vi "simpleInterpreter.vi"() -> ()   [LabVIEW 2011]
uses:
  <vilib>/Utility/inputDevices.llb/keyboardAcquire.vi
panel:
  out "error out":errorcluster
  out "lua_State *L":u64
  out "lua_State *print thread":u64
  in  "status refrash":bool
  in  "command refrash":bool
  out "stack":i32
  out "LoadBufferStatus":i32(ring) items=["LUA_OK", "LUA_YIELD", "LUA_ERRRUN", "LUA_ERRSYNTAX", "LUA_ERRMEM", "LUA_ERRGCMM", "LUA_ERRERR"]
  out "PcallStatus":i32(ring) items=["LUA_OK", "LUA_YIELD", "LUA_ERRRUN", "LUA_ERRSYNTAX", "LUA_ERRMEM", "LUA_ERRGCMM", "LUA_ERRERR"]
  in  "停止":bool
  in  "command(ctrl+enter)":string
  out "status":string
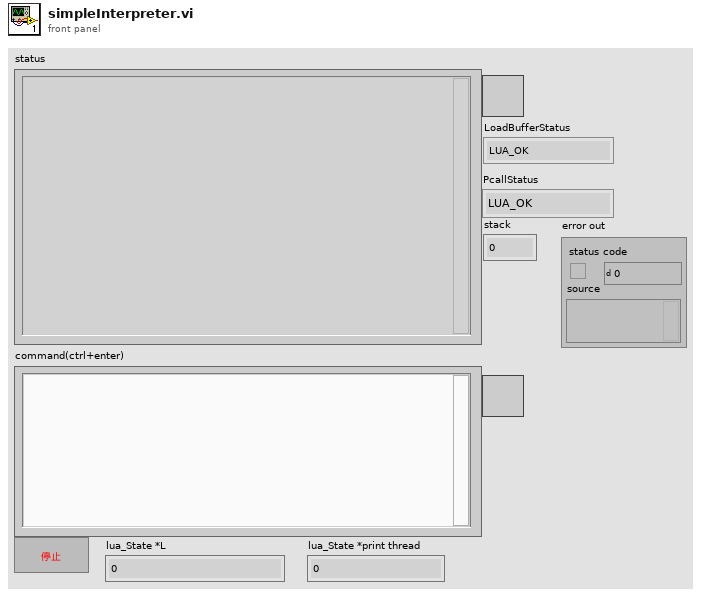
[diagram p1: front panel]
types:
  T1 = enum16{"0", "1", "2", "3", "4", "5", "6", "7", "8", "9", "A", "B", "C", "D", "E", "F", "G", "H", "I", "J", "K", "L", "M", "N", "O", "P", "Q", "R", "S", "T", "U", "V", "W", "X", "Y", "Z", "F1", "F2", "F3", "F4", "F5", "F6", "F7", "F8", "F9", "F10", "F11", "F12", "F13", "F14", "F15", "ADD", "BACK", "BACKSLASH", "CAPITAL", "COMMA", "DECIMAL", "DELETE", "DIVIDE", "DOWN", "END", "EQUALS", "ESCAPE", "GRAVE (`)", "HOME", "INSERT", "LBRACKET", "LCONTROL", "LEFT", "L ALT", "LSHIFT", "LWIN", "MINUS", "MULTIPLY", "NEXT", "NUMLOCK", "NUMPAD_0", "NUMPAD_1", "NUMPAD_2", "NUMPAD_3", "NUMPAD_4", "NUMPAD_5", "NUMPAD_6", "NUMPAD_7", "NUMPAD_8", "NUMPAD_9", "PAUSE", "PERIOD", "PRIOR (PG UP)", "RBRACKET", "RCONTROL", "RETURN", "RIGHT", "R ALT", "RSHIFT", "RWIN", "SCROLL", "SEMICOLON", "SLASH", "SPACE", "SUBTRACT", "TAB", "UP", "ENTER (num pad)", "' (quote)"}[]
  T2 = enum16{"0", "1", "2", "3", "4", "5", "6", "7", "8", "9", "A", "B", "C", "D", "E", "F", "G", "H", "I", "J", "K", "L", "M", "N", "O", "P", "Q", "R", "S", "T", "U", "V", "W", "X", "Y", "Z", "F1", "F2", "F3", "F4", "F5", "F6", "F7", "F8", "F9", "F10", "F11", "F12", "F13", "F14", "F15", "ADD", "BACK", "BACKSLASH", "CAPITAL", "COMMA", "DECIMAL", "DELETE", "DIVIDE", "DOWN", "END", "EQUALS", "ESCAPE", "GRAVE (`)", "HOME", "INSERT", "LBRACKET", "LCONTROL", "LEFT", "L ALT", "LSHIFT", "LWIN", "MINUS", "MULTIPLY", "NEXT", "NUMLOCK", "NUMPAD_0", "NUMPAD_1", "NUMPAD_2", "NUMPAD_3", "NUMPAD_4", "NUMPAD_5", "NUMPAD_6", "NUMPAD_7", "NUMPAD_8", "NUMPAD_9", "PAUSE", "PERIOD", "PRIOR (PG UP)", "RBRACKET", "RCONTROL", "RETURN", "RIGHT", "R ALT", "RSHIFT", "RWIN", "SCROLL", "SEMICOLON", "SLASH", "SPACE", "SUBTRACT", "TAB", "UP", "ENTER (num pad)", "' (quote)"}
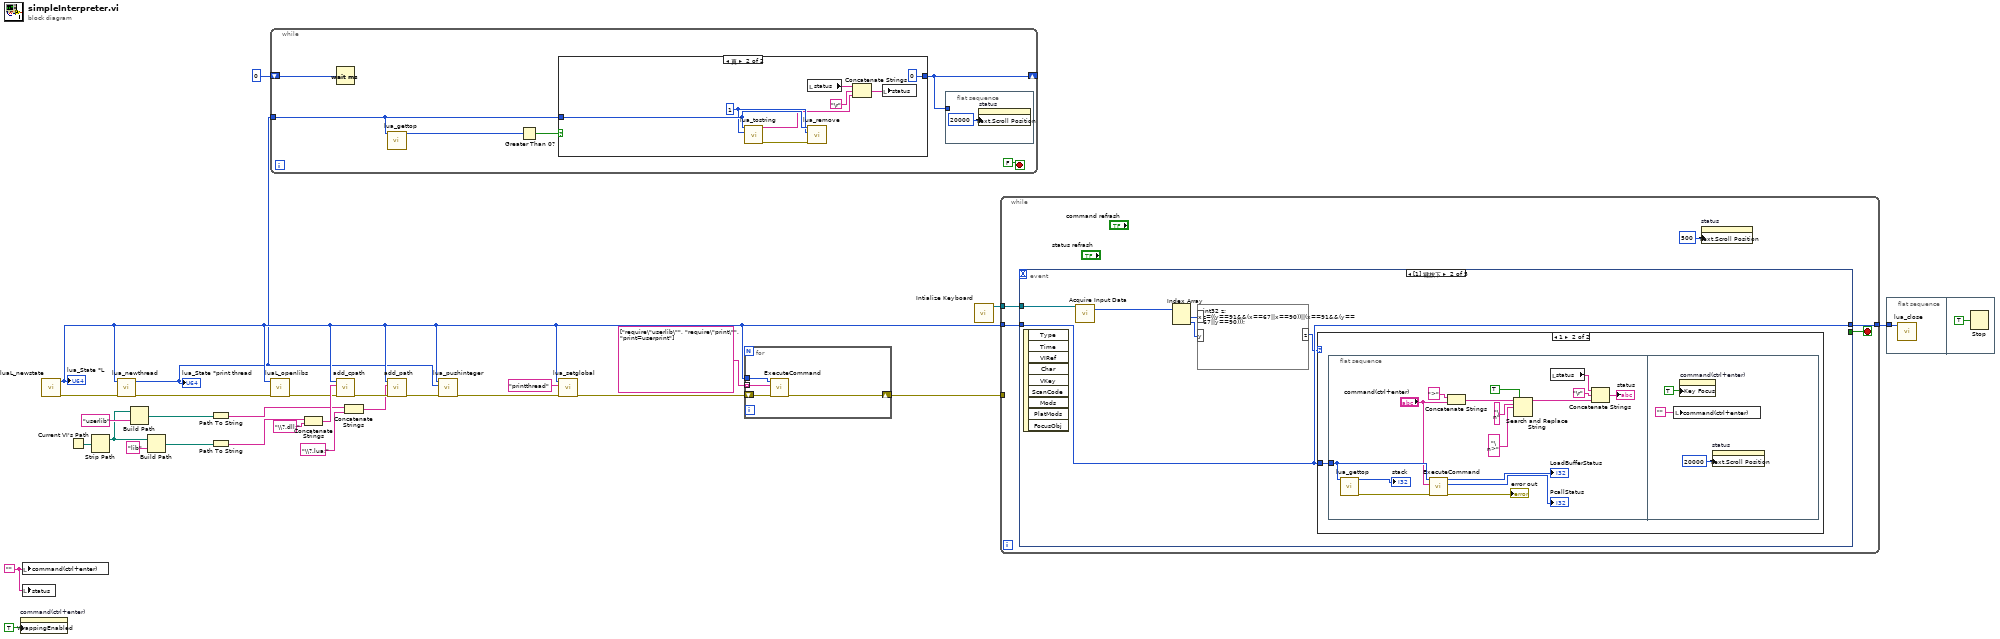
[diagram p0: block diagram]
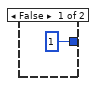
[diagram p2: hidden frame]
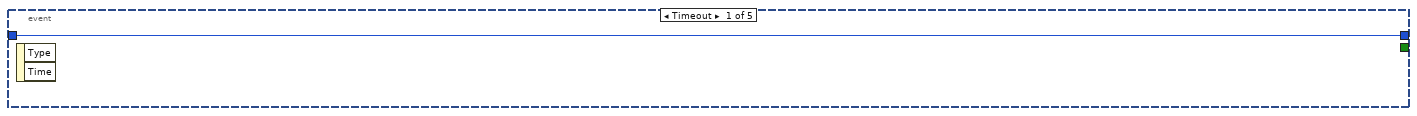
[diagram p3: hidden frame]
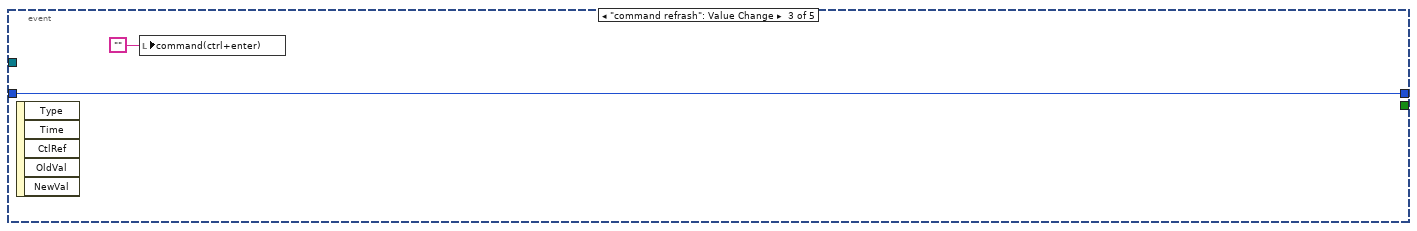
[diagram p5: hidden frame]
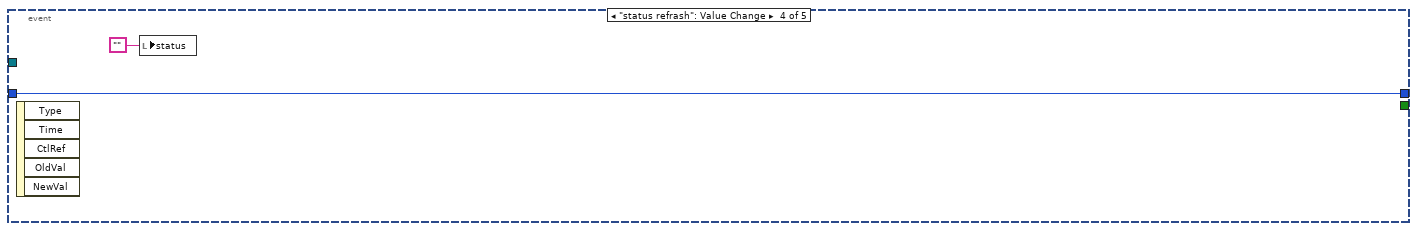
[diagram p6: hidden frame]
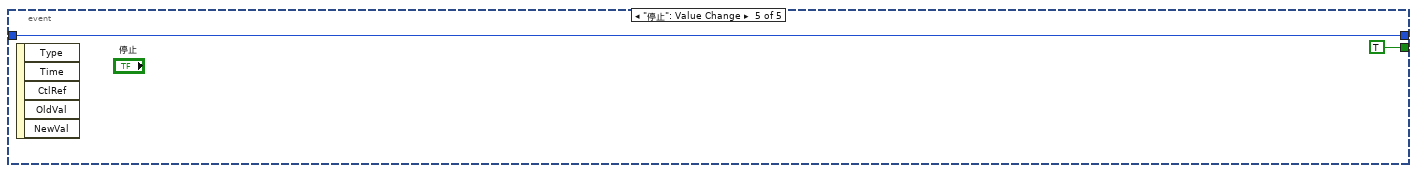
[diagram p7: hidden frame]
diagram:
  w29 = ""
  n1 = property on="command(ctrl+enter)" class="Str"("WrappingEnabled"=TRUE ("启用自动换行")) -> ()  [unwired: 2 in, 2 out]
  n2 = local write "command(ctrl+enter)"(w29) -> ()
  n3 = local write "status"(w29) -> ()
  n4 = call "luaL_newstate.vi"() -> ("error out"=w13:errorcluster, "lua_State *luaL_newstate"=w5:u64)  [unwired: 10 in]
  "lua_State *L" <- w5
  n5 = Current VI's Path() -> (path=w26:path)
  n6 = Strip Path(path=w26) -> (stripped path=w17:path)  [unwired: 1 out]
  n7 = call "lua_newthread.vi"("error in"=w13, "lua_State *L"=w5) -> ("error out"=w12:errorcluster, "lua_State *lua_newthread"=w2:u64)  [unwired: 8 in]
  "lua_State *print thread" <- w2
  n8 = Build Path(base path=w17, name or relative path="userlib" ("名称或相对路径")) -> (appended path=w24:path)
  n9 = Build Path(base path=w17, name or relative path="lib" ("名称或相对路径")) -> (appended path=w15:path)
  n10 = Path To String(path=w24) -> (string=w19:string)
  n11 = Path To String(path=w15) -> (string=w14:string)
  n12 = while {
    tunnel: w2 -> [w33]
    shift-right: [w30] -> _
    shift-left: u32 0 ("等待时间（毫秒）") -> [w31]
    stop <- FALSE stop-if-true
    n13 = Wait (ms)(milliseconds to wait=w31) -> ()  [unwired: 1 out]
    n14 = call "lua_gettop.vi"("lua_State *L"=w33) -> ("lua_gettop"=w34:i32)  [unwired: 9 in, 1 out]
    n15 = Greater Than 0?(x=w34) -> (x > 0?=w32:bool)
    n16 = case shown="真" w32 {
      tunnel: w33 -> [_ w43]
      tunnel: [u32 1 ("等待时间（毫秒）") u32 0 ("等待时间（毫秒）")] -> w30
      frame False {
      }
      frame True {
        w42 = 1 ("index")
        n17 = call "lua_tostring.vi"("index"=w42, "lua_State *L"=w43) -> ("error out"=w44:errorcluster, "constant string"=w38:string)  [unwired: 8 in]
        n18 = local read "status"() -> (w40:string)
        n19 = call "lua_remove.vi"("error in"=w44, "int index"=w42, "lua_State *L"=w43) -> ()  [unwired: 8 in, 1 out]
        n20 = Concatenate Strings(w40, "\r", w38) -> (w41:string)
        n21 = local write "status"(w41) -> ()
      }
    }
    n22 = flat-sequence {
      tunnel: w30 -> [_]
      frame #0 {
        n23 = property on="status" class="Str"("Text.Scroll Position"=u32 20000 ("文本.滚动条位置")) -> ()  [unwired: 2 in, 2 out]
      }
    }
  }
  n24 = call "luaL_openlibs.vi"("error in"=w12, "lua_State *L"=w5) -> ("error out"=w11:errorcluster)  [unwired: 9 in]
  n25 = Concatenate Strings(w14, "\\?.dll;" ("字符串")) -> (w22:string)
  n26 = call "add_cpath.vi"("error in"=w11, "string"=w22, "lua_State *L"=w5) -> ("error out"=w21:errorcluster)  [unwired: 8 in]
  n27 = Concatenate Strings(w19, "\\?.lua;" ("字符串")) -> (w18:string)
  n28 = call "add_path.vi"("error in"=w21, "string"=w18, "lua_State *L"=w5) -> ("error out"=w7:errorcluster)  [unwired: 8 in]
  n29 = call "lua_pushinteger.vi"("error in"=w7, "lua_Integer n"=w2, "lua_State *L"=w5) -> ("error out"=w6:errorcluster)  [unwired: 8 in]
  n30 = call "lua_setglobal.vi"("error in"=w6, "s"="printthread" ("const char *k"), "lua_State *L"=w5) -> ("error out"=w3:errorcluster)  [unwired: 8 in]
  n31 = for {
    shift-right: [w48] -> w9
    shift-left: w3 -> [w49]
    tunnel: w5 -> [w47]
    tunnel: string[] ["require\"userlib\"", "require\"print\"", "print=userprint"] -> [w46] mode=indexing
    n32 = call "ExecuteCommand.vi"("error in"=w49, "command(ctrl+enter)"=w46, "lua_State *luaL_newstate"=w47) -> ("error out"=w48:errorcluster)  [unwired: 6 in, 2 out]
  }
  n33 = call <vilib>:"Intialize Keyboard.vi"() -> ("device ID"=w27:refnum<k1>)  [unwired: 10 in, 1 out]
  n34 = while {
    tunnel: w5 -> [w54]
    tunnel: [w52] -> w1
    tunnel: w27 -> [w51]
    tunnel: w9 -> [_]
    stop <- w53 stop-if-true
    n35 = event shown="[1] 键按下" {
      selector: _ -> [_ _ _ _ _]
      dyn-events: _ -> [_ _ _ _ _]
      timeout: _ -> [_ _ _ _ _]
      tunnel: w54 -> [w55 w61 w82 w84 w86]
      tunnel: [_ _ _ _ TRUE ("停止 2")] -> w53
      tunnel: [w55 w61 w82 w84 w86] -> w52
      tunnel: w51 -> [_ w60 _ _ _]
      event Timeout {
        n36 = event-data() -> ()  [unwired: 1 in, 2 out]
      }
      event Key Down {
        n37 = event-data() -> ()  [unwired: 1 in, 9 out]
        n38 = call-poly <vilib>:"Acquire Input Data.vi"("device ID"=w60) -> ("keys pressed"=w59:T1)  [unwired: 16 in, 2 out]
        n39 = Index Array(array=w59) -> (element #1=w58:T2, element #2=w57:T2)  [unwired: 2 in]
        n40 = formula code="int32 z;\nz=((y==91&&(x==67||x==90))||(x==91&&(y==67||y==90)));"("x"=w58, "y"=w57) -> ("z"=w56:i32)
        n41 = case shown="1" w56 {
          tunnel: w61 -> [_ w62]
          frame 0, Default {
          }
          frame 1 {
            n42 = flat-sequence {
              tunnel: w62 -> [w71]
              frame #0 {
                n43 = call "lua_gettop.vi"("lua_State *L"=w71) -> ("error out"=w72:errorcluster, "lua_gettop"=→"stack":i32)  [unwired: 9 in]
                n44 = call "ExecuteCommand.vi"("error in"=w72, "command(ctrl+enter)"="command(ctrl+enter)", "lua_State *luaL_newstate"=w71) -> ("error out"=→"error out":errorcluster, "thread status 2"=→"PcallStatus":i32, "thread status"=→"LoadBufferStatus":i32)  [unwired: 6 in]
                n45 = Concatenate Strings(">", "command(ctrl+enter)") -> (w67:string)
                n46 = Search and Replace String(replace all?=TRUE ("替换全部？(F)"), input string=w67, search string="\n" ("搜索字符串"), replace string="\n>" ("替换字符串(\"\")")) -> (result string=w63:string)  [unwired: 4 in, 3 out]
                n47 = local read "status"() -> (w77:string)
                n48 = Concatenate Strings(w77, "\r", w63) -> (→"status":string)
              }
              frame #1 {
                n49 = local write "command(ctrl+enter)"("") -> ()
                n50 = property on="command(ctrl+enter)" class="Str"("Key Focus"=TRUE ("键选中")) -> ()  [unwired: 2 in, 2 out]
                n51 = property on="status" class="Str"("Text.Scroll Position"=u32 20000 ("文本.滚动条位置")) -> ()  [unwired: 2 in, 2 out]
              }
            }
          }
        }
      }
      event "command refrash": Value Change {
        n52 = event-data() -> ()  [unwired: 1 in, 5 out]
        n53 = local write "command(ctrl+enter)"("") -> ()
      }
      event "status refrash": Value Change {
        n54 = event-data() -> ()  [unwired: 1 in, 5 out]
        n55 = local write "status"("") -> ()
      }
      event "停止": Value Change {
        n56 = event-data() -> ()  [unwired: 1 in, 5 out]
      }
    }
    n57 = property on="status" class="Str"("Text.Scroll Position"=u32 500 ("文本.滚动条位置")) -> ()  [unwired: 2 in, 2 out]
  }
  n58 = flat-sequence {
    tunnel: w1 -> [w88]
    frame #0 {
      n59 = call "lua_close.vi"("lua_State *L"=w88) -> ()  [unwired: 10 in, 1 out]
    }
    frame #1 {
      n60 = Stop(stop? (T)=TRUE ("停止？(T)")) -> ()
    }
  }
